vi "Update Speaker Selection.vi"(0 "states in":T1[](array[typedef]), 5 "index":i32, 7 "sel speak":i32, 9 "Shift":bool) -> (4 "states out":T1[](array[typedef]))   [LabVIEW 2015, in "SAC Config.xctl"]
uses:
  SAC Config.xctl
  Speaker State.ctl
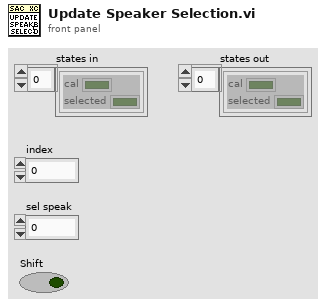
[diagram p1: front panel]
types:
  T1 = typedef "SAC Config.xctl/Speaker State.ctl" = cluster{"cal":bool, "selected":bool}
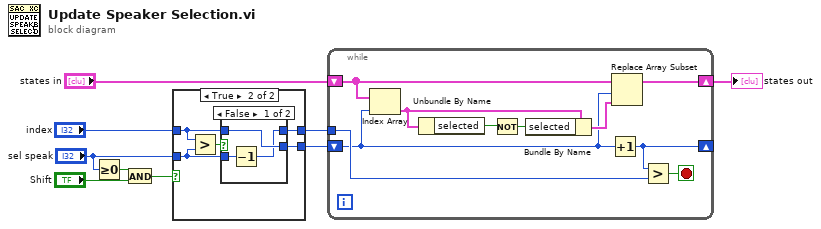
[diagram p0: block diagram]
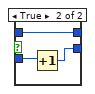
[diagram p3: hidden frame]
diagram:
  n1 = Greater Or Equal To 0?(x="sel speak") -> (x >= 0?=w6:bool)
  n2 = And(x=w6, y="Shift") -> (x .and. y?=w7:bool)
  n3 = case shown="True" w7 {
    tunnel: "sel speak" -> [_ w13]
    tunnel: "index" -> [w10 w14]
    tunnel: [w10 w12] -> w3
    tunnel: [w10 w11] -> w4
    frame False {
    }
    frame True {
      n4 = Greater?(x=w14, y=w13) -> (0:w15:bool)
      n5 = case shown="False" w15 {
        tunnel: w14 -> [w17 w20]
        tunnel: w13 -> [w18 w21]
        tunnel: [w17 w19] -> w12
        tunnel: [w16 w20] -> w11
        frame False {
          n6 = Decrement(x=w18) -> (x-1=w16:i32)
        }
        frame True {
          n7 = Increment(x=w21) -> (x+1=w19:i32)
        }
      }
    }
  }
  n8 = while {
    tunnel: w4 -> [w30]
    shift-right: [w31] -> _
    shift-left: w3 -> [w22]
    shift-right: [w24] -> w1
    shift-left: "states in" -> [w25]
    stop <- w29 stop-if-true
    n9 = Index Array(array=w25, index=w22) -> (element=w26:T1)
    n10 = Unbundle By Name(w26) -> ("selected"=w28:bool)
    n11 = Not(x=w28) -> (.not. x?=w27:bool)
    n12 = Bundle By Name(cluster=w26, "selected"=w27) -> (w23:T1)
    n13 = Increment(x=w22) -> (x+1=w31:i32)
    n14 = Replace Array Subset(array=w25, new element=w23, index=w22) -> (w24:T1[])
    n15 = Greater?(x=w31, y=w30) -> (0:w29:bool)
  }
  "states out" <- w1
